vi "Get Active Line Channel Name.vi"(8 "error in (no error)":errorcluster, 11 "Pairing Tab Refs":T1) -> (0 "error out":errorcluster, 2 "Channel Name":string)   [LabVIEW 2015, in "E2E Tag Exchange editor node.lvclass"]
uses:
  E2E Tag Exchange editor node.lvclass
  Tag Exchange Tab References.ctl
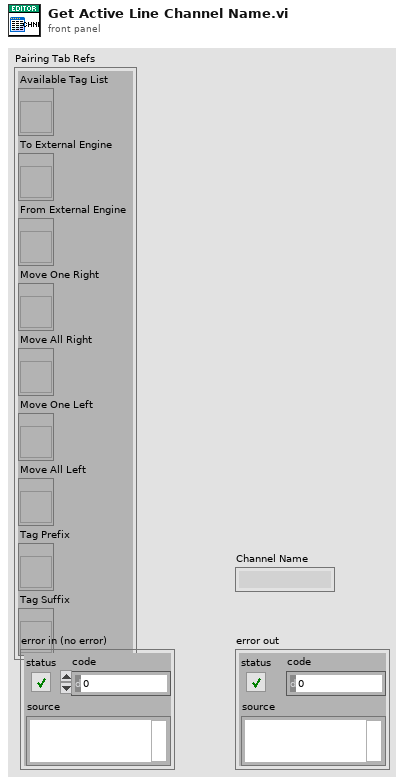
[diagram p1: front panel]
types:
  T1 = typedef "E2E Tag Exchange editor node.lvclass/Tag Exchange Tab References.ctl" = cluster{"Available Tag List":refnum<vi>, "To External Engine":refnum<vi>, "From External Engine":refnum<vi>, "Move One Right":refnum<vi>, "Move All Right":refnum<vi>, "Move One Left":refnum<vi>, "Move All Left":refnum<vi>, "Tag Prefix":refnum<vi>, "Tag Suffix":refnum<vi>}
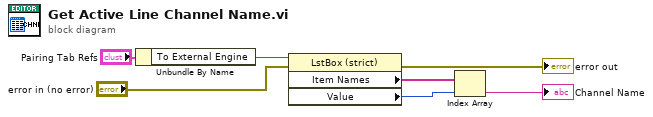
[diagram p0: block diagram]
diagram:
  n1 = Unbundle By Name("Pairing Tab Refs") -> ("To External Engine"=w6:refnum<vi>)
  n2 = property class="LstBox (strict)"(reference=w6, error in="error in (no error)") -> (error out=→"error out":errorcluster, "Item Names"=w5:string[], "Value"=w4:i32)  [unwired: 1 out]
  n3 = Index Array(array=w5, index=w4) -> (element=→"Channel Name":string)
